vi "GV-CursorZoomHorStart.vi"(6 "time":string, 7 "Gviewer in":refnum<class "Gviewer.lvclass">, 8 "error in (no error)":errorcluster, 10 "Pos":cluster{"x":i16, "y":i16}, 11 "pict in":picture) -> (0 "error out":errorcluster, 3 "pict out":picture)   [LabVIEW 2020, in "Gviewer.lvclass"]
doc: "Andre Koelewijn, 8 may 2021\n\nDefine starting point for Horizontal Window Zoom.\nThis function allows zooming for one selected TAG or all TAGs"
uses:
  Gviewer.lvclass
  Gviewer.lvclass/Gviewer.ctl
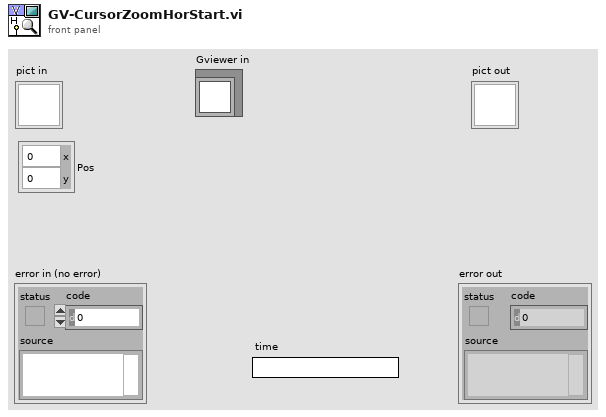
[diagram p1: front panel]
types:
  T1 = cluster{"horizontal":enum16{"left", "center", "right"}, "vertical":enum16{"top", "center", "bottom"}}
  T2 = cluster{"Width":u16, "Style":enum32{"Solid", "Dash", "Dot", "DashDot", "DashDotDot"}}
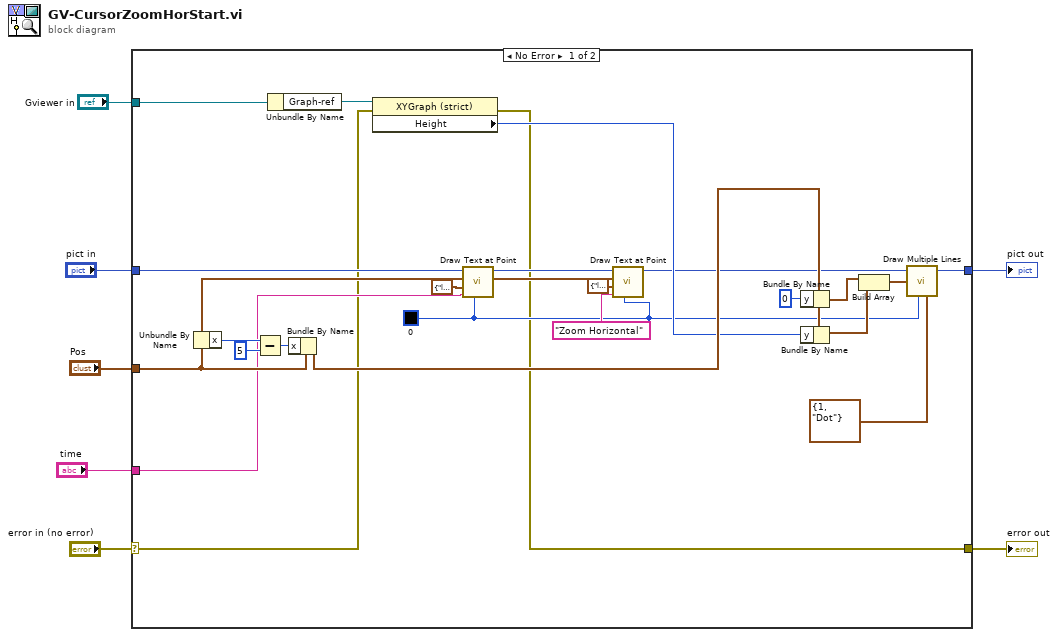
[diagram p0: block diagram]
diagram:
  n1 = case shown="No Error" "error in (no error)" {
    selector: "error in (no error)" -> [w9 w33]
    tunnel: [w8 w33] -> w6
    tunnel: "pict in" -> [w15 w32]
    tunnel: [w10 w32] -> w4
    tunnel: "Pos" -> [w16 _]
    tunnel: "Gviewer in" -> [w24 _]
    tunnel: "time" -> [w12 _]
    frame No Error {
      w11 = u32 0 ("Color")
      n2 = Unbundle By Name(w16) -> ("x"=w23:i16)
      n3 = Subtract(x=w23, y=i16 5) -> (x-y=w21:i16)
      n4 = Unbundle By Name(w24) -> ("Graph-ref"=w18:refnum<vi>)
      n5 = Bundle By Name(cluster=w16, "x"=w21) -> (w19:cluster{"x":i16, "y":i16})
      n6 = property class="XYGraph (strict)"(reference=w18, error in=w9) -> (error out=w8:errorcluster, "Height"=w17:u32)  [unwired: 1 out]
      n7 = call <vilib>:"Draw Text at Point.vi"("text color(black)"=w11, "text"=w12, "alignment(left, top)"=T1 {"horizontal"=enum."left", "vertical"=enum."top"}, "origin"=w16, "picture"=w15) -> ("new picture"=w14:picture)  [unwired: 5 in, 1 out]
      n8 = call <vilib>:"Draw Text at Point.vi"("text color(black)"=w11, "text"="Zoom Horizontal", "alignment(left, top)"=T1 {"horizontal"=enum."left", "vertical"=enum."bottom"}, "origin"=w16, "picture"=w14) -> ("new picture"=w13:picture)  [unwired: 5 in, 1 out]
      n9 = Bundle By Name(cluster=w19, "y"=i16 0 ("x")) -> (w28:cluster{"x":i16, "y":i16})
      n10 = Bundle By Name(cluster=w19, "y"=w17) -> (w30:cluster{"x":i16, "y":i16})
      n11 = Build Array(w28, w30) -> (w31:cluster{"x":i16, "y":i16}[])
      n12 = call <vilib>:"Draw Multiple Lines.vi"("picture"=w13, "line endpoints"=w31, "color(black)"=w11, "pen"=T2 {"Width"=1, "Style"=enum."Dot"}) -> ("new picture"=w10:picture)  [unwired: 5 in]
    }
    frame Error {
    }
  }
  "error out" <- w6
  "pict out" <- w4
